vi "Undefined State Notification.vi"(8 "error in":errorcluster, 10 "Undefined state":string, 11 "Rename in":refnum<class "Rename.lvclass">) -> (0 "error out":errorcluster, 3 "Rename out":refnum<class "Rename.lvclass">)   [LabVIEW 2015, in "Generic Module Library.lvlib" / "Template G_Module.lvlib" / "Rename.lvclass"]
uses:
  Rename.lvclass
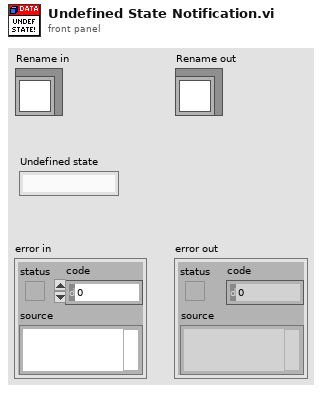
[diagram p1: front panel]
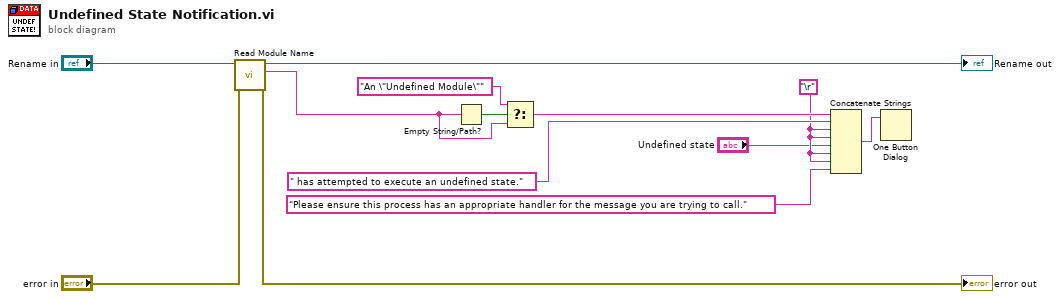
[diagram p0: block diagram]
diagram:
  w3 = "\r"
  n1 = call-dynamic "Read Module Name.vi"("error in (no error)"="error in", "Rename in"="Rename in") -> ("error out"=→"error out":errorcluster, "Module Name"=w5:string, "Rename out"=→"Rename out":refnum<class "Rename.lvclass">)  [unwired: 7 in]
  n2 = Empty String/Path?(string/path=w5) -> (empty?=w9:bool)
  n3 = Select(t="An \"Undefined Module\"", s=w9, f=w5) -> (s? t:f=w7:string)
  n4 = Concatenate Strings(w7, " has attempted to execute an undefined state.", w3, w3, "Undefined state", w3, w3, "Please ensure this process has an appropriate handler for the message you are trying to call.") -> (w10:string)
  n5 = One Button Dialog(message=w10) -> ()  [unwired: 1 in, 1 out]
